vi "MainLossy EnQueue.vi"(8 "error in":errorcluster, 11 "States":T1) -> (0 "error out":errorcluster)   [LabVIEW 2022 SP3]
uses:
  Type Def/MainStates Cluster.ctl
  Type Def/MainStates.ctl
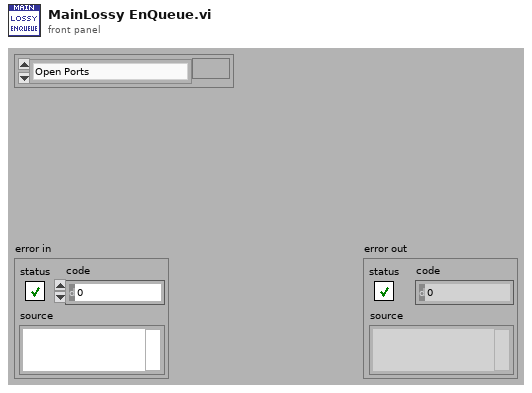
[diagram p1: front panel]
types:
  T1 = typedef "MainStates Cluster.ctl" = cluster{"States":T2, "Data":variant}
  T2 = typedef "MainStates.ctl" = enum16{"Open Ports", "Close Ports", "Main", "Settings", "Voltaje", "Probe", "Lenguaje", "Callibration", "Exit", "Voltage Test", "Test 2", "End test"}
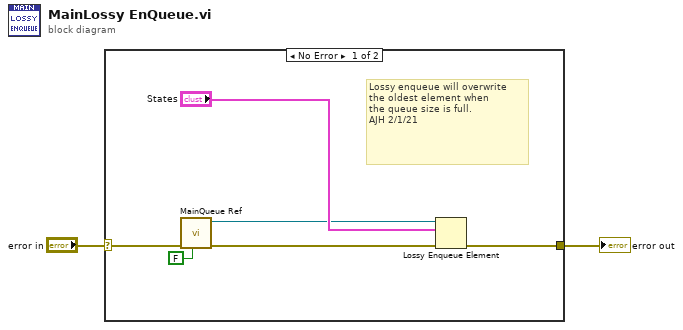
[diagram p0: block diagram]
diagram:
  n1 = case shown="No Error" "error in" {
    selector: "error in" -> [w7 w9]
    tunnel: [w5 w9] -> w1
    frame No Error {
      # "Lossy enqueue will overwrite\nthe oldest element when\nthe queue size is full.   \nAJH 2/1/21"
      n2 = call "MainQueue Ref.vi"("Write:T/Read:(F)"=FALSE ("Write:T/Read:F"), "error in"=w7) -> ("error out"=w6:errorcluster, "queue out"=w3:refnum<queue>)  [unwired: 8 in]
      n3 = Lossy Enqueue Element(queue=w3, element="States", error in (no error)=w6) -> (error out=w5:errorcluster)  [unwired: 3 out]
    }
    frame Error {
    }
  }
  "error out" <- w1
